vi "ex_7.vi"() -> ()   [LabVIEW 2020]
panel:
  out "Palindrome":bool
  in  "Text":string
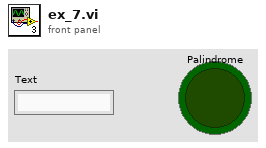
[diagram p1: front panel]
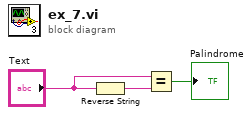
[diagram p0: block diagram]
diagram:
  n1 = Reverse String(1:"Text") -> (0:w3:string)
  n2 = Equal?(x="Text", y=w3) -> (x = y?=→"Palindrome":bool)
